vi "License Request Form.vi"(8 "Error in (no error)":errorcluster) -> (0 "Error out":errorcluster)   [LabVIEW 2021]
uses:
  Controls/License Request Form States.ctl
  Controls/License Request Form.ctl
panel:
  in  "Cancel":bool
  in  "Add License File":bool
  in  "Generate Info File":bool
  in  "Phone":string
  in  "Email":string
  in  "Organization Name":string
  in  "Name":string
  # "License Request Form"
  # "Note: Send the Generated file to license@karmainnovations.com"
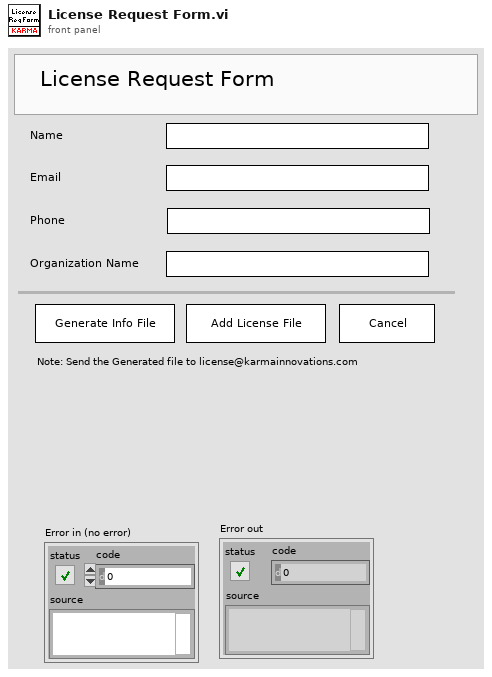
[diagram p1: front panel]
types:
  T1 = typedef "License Request Form.ctl" = cluster{"Name":string, "Email":string, "Phone":string, "Computer ID":string, "Org Name":string, "Created Date":string, "Sensor ID":string}
  T2 = typedef "License Request Form States.ctl" = enum16{"Poll", "Initialize", "Update Display", "Generate Info File", "Add License File", "Error", "Exit"}
  T3 = typedef "Paths.ctl" = cluster{"Configuration":path, "Event Logs":path, "Error Logs":path, "Macros":path, "Camera Settings":path, "Settings.ini":path, "UserInfo.bin":path, "TimeStamp File":path, "FileCounter.txt":path, "FFC Images":path, "Calibration.txt":path, "Bright Images - FFC":path, "Dark Images - FFC":path, "Last FFC Time File":path, "BG Subtraction Folder":path, "BG Mask":path, "LUTs Folder":path}
  T4 = enum32{"invalid app kind", "Development System", "Run Time System", "Student Edition", "Embedded LabVIEW", "Evaluation", "Custom"}
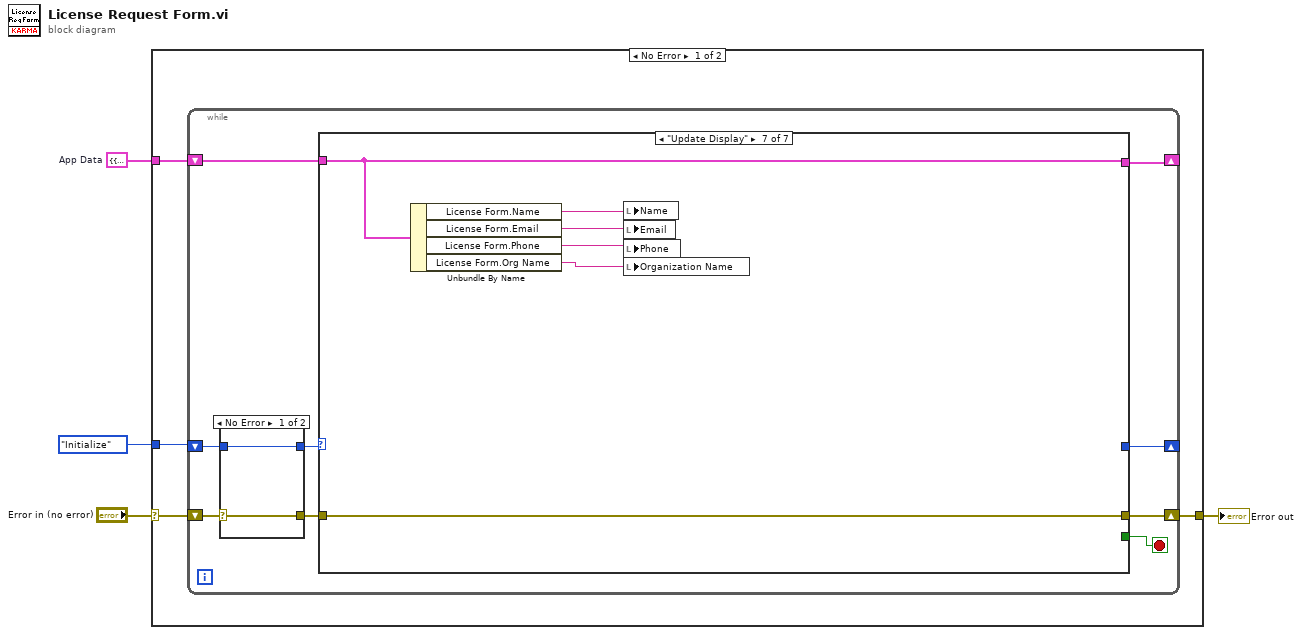
[diagram p0: block diagram]
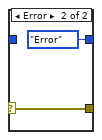
[diagram p2: hidden frame]
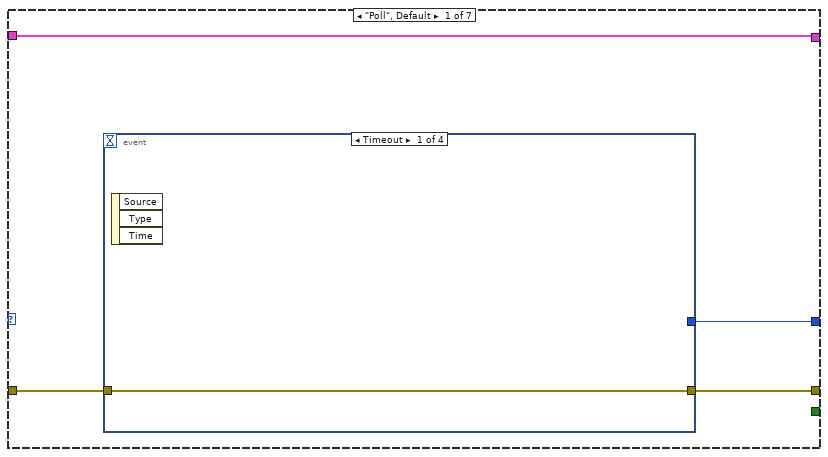
[diagram p3: hidden frame]
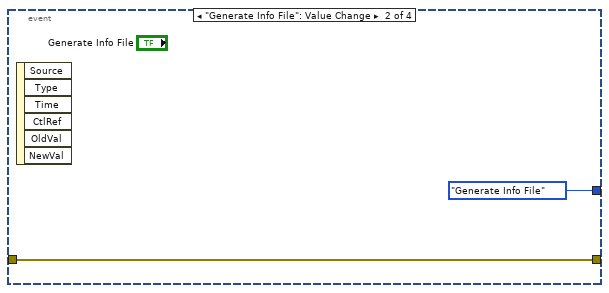
[diagram p4: hidden frame]
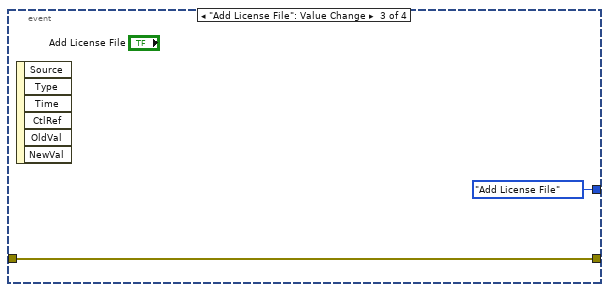
[diagram p5: hidden frame]
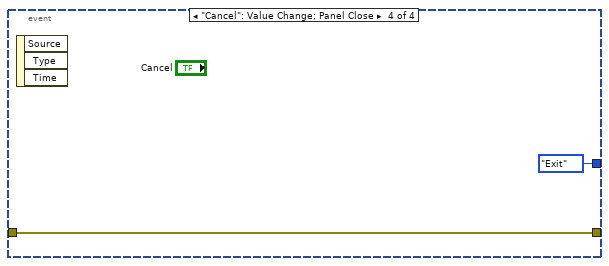
[diagram p6: hidden frame]
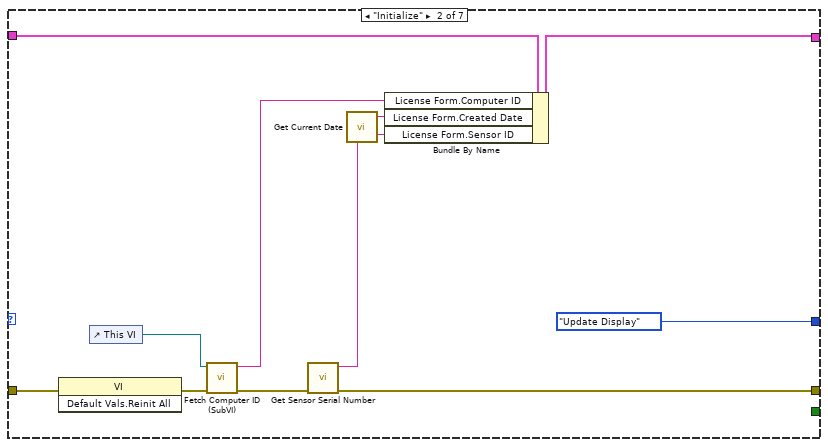
[diagram p7: hidden frame]
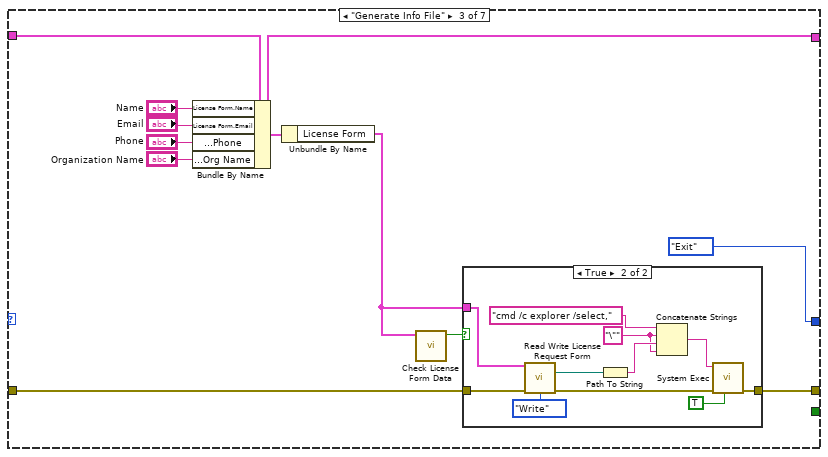
[diagram p8: hidden frame]
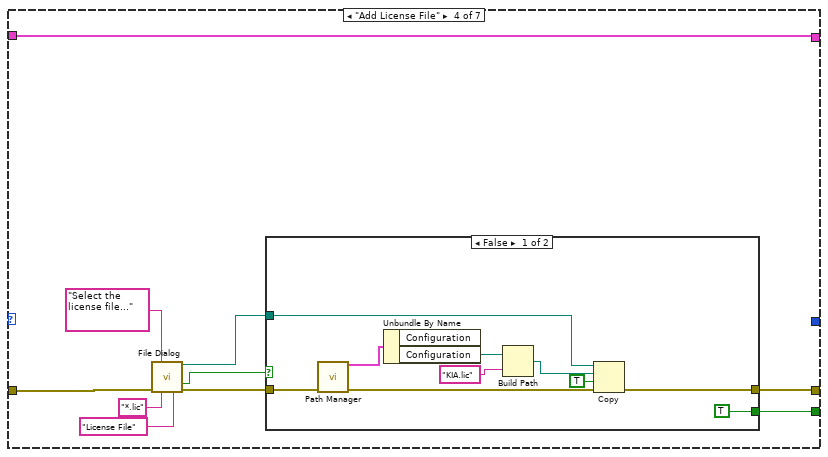
[diagram p10: hidden frame]
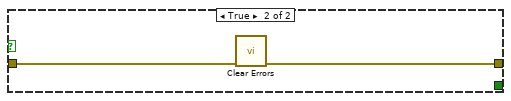
[diagram p11: hidden frame]
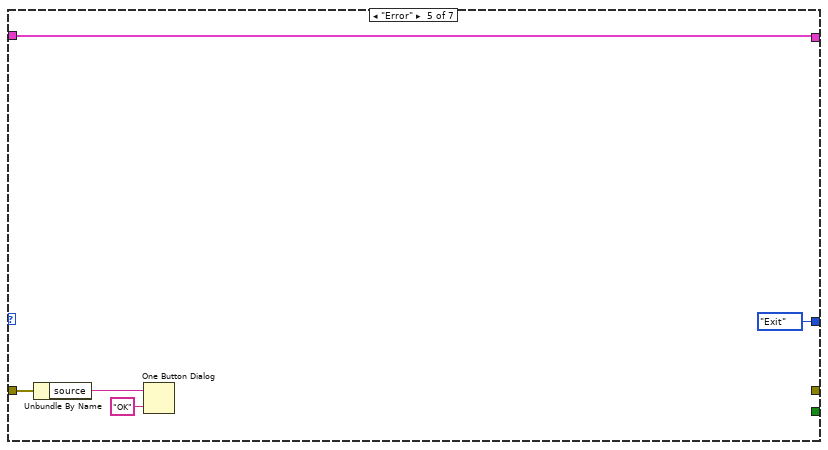
[diagram p12: hidden frame]
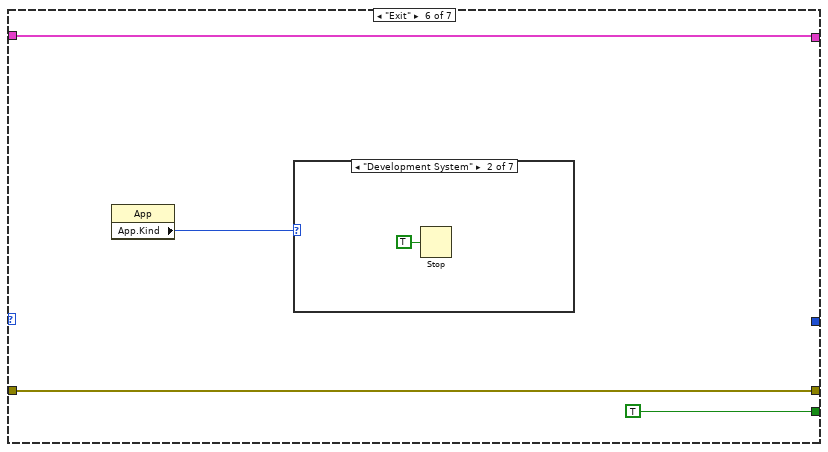
[diagram p13: hidden frame]
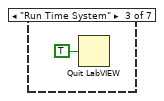
[diagram p15: hidden frame]
diagram:
  w1 = cluster{"License Form":T1} {"License Form"={"Name"="", "Email"="", "Phone"="", "Computer ID"="", "Org Name"="", "Created Date"="", "Sensor ID"=""}}  # App Data
  n1 = case shown="No Error" "Error in (no error)" {
    selector: "Error in (no error)" -> [w8 w106]
    tunnel: [w7 w106] -> w3
    tunnel: License_Request_Form_States."Initialize" -> [w6 _]
    tunnel: w1 -> [w5 _]
    frame No Error {
      n2 = while {
        shift-right: [w15] -> _
        shift-left: w5 -> [w16]
        shift-right: [w14] -> _
        shift-left: w6 -> [w11]
        shift-right: [w17] -> w7
        shift-left: w8 -> [w12]
        stop <- w13 stop-if-true
        n3 = case shown="No Error" w12 {
          selector: w12 -> [w18 w20]
          tunnel: w11 -> [w19 _]
          tunnel: [w19 License_Request_Form_States."Error"] -> w10
          tunnel: [w18 w20] -> w9
          frame No Error {
          }
          frame Error {
          }
        }
        n4 = case shown="\"Update Display\"" w10 {
          tunnel: w9 -> [w25 w38 w48 w75 w91 w97 w100]
          tunnel: [w24 w34 w47 w69 _ w97 w100] -> w17
          tunnel: [w22 w42 w49 w76 w93 w96 w101] -> w15
          tunnel: w16 -> [w22 w43 w50 w76 w93 w96 w101]
          tunnel: [w23 License_Request_Form_States."Update Display" License_Request_Form_States."Exit" _ License_Request_Form_States."Exit" _ _] -> w14
          tunnel: [_ _ _ w67 _ TRUE _] -> w13
          frame "Poll", Default {
            n5 = event shown="[0] Timeout" {
              selector: _ -> [_ _ _ _]
              dyn-events: _ -> [_ _ _ _]
              timeout: _ -> [_ _ _ _]
              tunnel: w25 -> [w26 w27 w29 w31]
              tunnel: [w26 w27 w29 w31] -> w24
              tunnel: [_ License_Request_Form_States."Generate Info File" License_Request_Form_States."Add License File" License_Request_Form_States."Exit"] -> w23
              event Timeout {
                n6 = event-data() -> ()  [unwired: 1 in, 3 out]
              }
              event "Generate Info File": Value Change {
                n7 = event-data() -> ()  [unwired: 1 in, 6 out]
              }
              event "Add License File": Value Change {
                n8 = event-data() -> ()  [unwired: 1 in, 6 out]
              }
              event "Cancel": Value Change; Panel Close {
                n9 = event-data() -> ()  [unwired: 1 in, 3 out]
              }
            }
          }
          frame "Initialize" {
            n10 = invoke class="VI" method="Default Vals.Reinit All"(error in=w38) -> (error out=w37:errorcluster)  [unwired: 2 in, 2 out]
            n11 = control-ref of="This VI"() -> (w36:refnum<vi>)
            n12 = call "Fetch Computer ID (SubVI).vi"("Error in (no error)"=w37, "VI Reference"=w36) -> ("Error out"=w35:errorcluster, "Computer ID"=w41:string)  [unwired: 8 in]
            n13 = call "Get Sensor Serial Number.vi"("Error in (no error)"=w35) -> ("Error out"=w34:errorcluster, "Serial Number"=w33:string)  [unwired: 9 in]
            n14 = call "Get Current Date.vi"() -> ("Date String"=w40:string)  [unwired: 8 in]
            n15 = Bundle By Name(cluster=w43, "License Form.Computer ID"=w41, "License Form.Created Date"=w40, "License Form.Sensor ID"=w33) -> (w42:cluster{"License Form":T1})
          }
          frame "Generate Info File" {
            n16 = Bundle By Name(cluster=w50, "License Form.Name"="Name", "License Form.Email"="Email", "License Form.Phone"="Phone", "License Form.Org Name"="Organization Name") -> (w49:cluster{"License Form":T1})
            n17 = Unbundle By Name(w49) -> ("License Form"=w46:T1)
            n18 = call "Check License Form Data.vi"("License Form"=w46) -> ("Data Valid (F)"=w45:bool)  [unwired: 9 in, 1 out]
            n19 = case shown="True" w45 {
              tunnel: w48 -> [w55 w66]
              tunnel: w46 -> [_ w64]
              tunnel: [w55 w62] -> w47
              frame False {
              }
              frame True {
                w59 = "\"" ("string")
                n20 = call "Read Write License Request Form.vi"("License Form"=w64, "Error in (no error)"=w66, "Operation"=enum16{"Write", "Read"}."Write") -> ("Info File Path"=w61:path, "Error out"=w63:errorcluster)  [unwired: 10 in, 1 out]
                n21 = Path To String(path=w61) -> (string=w60:string)
                n22 = Concatenate Strings("cmd /c explorer /select," ("string"), w59, w60, w59) -> (w56:string)
                n23 = call <vilib>:"System Exec.vi"("run minimized? (F)"=TRUE, "error in (no error)"=w63, "command line"=w56) -> ("error out"=w62:errorcluster)  [unwired: 5 in, 3 out]
              }
            }
          }
          frame "Add License File" {
            n24 = call "File Dialog"("prompt"="Select the license file...", "error in"=w75, "pattern (all files)"="*.lic", "pattern label"="License File") -> ("selected path"=w68:path, "cancelled"=w71:bool, "error out"=w70:errorcluster)  [unwired: 8 in, 1 out]
            n25 = case shown="False" w71 {
              tunnel: w70 -> [w84 w88]
              tunnel: [w86 w87] -> w69
              tunnel: w68 -> [w85 _]
              tunnel: [TRUE _] -> w67
              frame False {
                n26 = call "Path Manager.vi"("error in (no error)"=w84) -> ("Cluster"=w82:T3, "Error out"=w83:errorcluster)  [unwired: 13 in]
                n27 = Unbundle By Name(w82) -> ("Configuration"=w81:path)  [unwired: 1 out]
                n28 = Build Path(base path=w81, name or relative path="KIA.lic") -> (appended path=w79:path)
                n29 = Copy(8:w83, 9:TRUE ("overwrite (F)"), 10:w79, 11:w85) -> (0:w86:errorcluster)  [unwired: 1 in, 2 out]
              }
              frame True {
                n30 = call <vilib>:"Clear Errors.vi"("error in (no error)"=w88) -> ("error out"=w87:errorcluster)  [unwired: 5 in, 1 out]
              }
            }
          }
          frame "Error" {
            n31 = Unbundle By Name(w91) -> ("source"=w90:string)
            n32 = One Button Dialog(message=w90, button name ("OK")="OK") -> ()  [unwired: 1 out]
          }
          frame "Exit" {
            n33 = property class="App"() -> ("App.Kind"=w94:T4)  [unwired: 2 in, 2 out]
            n34 = case shown="\"Development System\"" w94 {
              frame "invalid app kind", Default {
              }
              frame "Development System" {
                n35 = Stop(stop? (T)=TRUE) -> ()
              }
              frame "Run Time System" {
                n36 = Quit LabVIEW(quit? (T)=TRUE) -> ()
              }
              frame "Student Edition" {
              }
              frame "Embedded LabVIEW" {
              }
              frame "Evaluation" {
              }
              frame "Custom" {
              }
            }
          }
          frame "Update Display" {
            n37 = Unbundle By Name(w101) -> ("License Form.Name"=w105:string, "License Form.Email"=w102:string, "License Form.Phone"=w103:string, "License Form.Org Name"=w104:string)
            n38 = local write "Name"(w105) -> ()
            n39 = local write "Email"(w102) -> ()
            n40 = local write "Phone"(w103) -> ()
            n41 = local write "Organization Name"(w104) -> ()
          }
        }
      }
    }
    frame Error {
    }
  }
  "Error out" <- w3
